vi "Read Error.vi"(11 "Result in":refnum<class "Result.lvclass">) -> (2 "Error":string, 3 "Result out":refnum<class "Result.lvclass">)   [LabVIEW 2018, in "InfluxDB Client.lvlib" / "Result.lvclass"]
uses:
  Result.lvclass
  Result.lvclass/Result.ctl
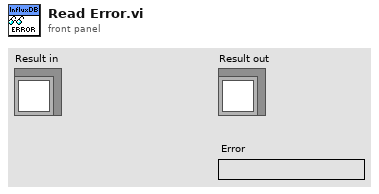
[diagram p1: front panel]
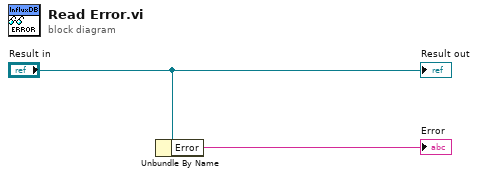
[diagram p0: block diagram]
diagram:
  n1 = Unbundle By Name("Result in") -> ("Error"=→"Error":string)
  "Result out" <- "Result in"
